vi "Remove_Child_Panel.vi"(8 "error in (no error)":errorcluster, 10 "Child_Panel in":refnum<class "Panel_Adaptive.lvclass">, 11 "Parent_Panel in":refnum<class "Panel2.lvclass">) -> (0 "error out":errorcluster, 1 "Status":bool, 2 "Child_Panel out":refnum<class "Panel_Interface.lvclass">[](array[class]), 3 "Parent_Panel out":refnum<class "Panel2.lvclass">, 4 "Child_Panel#":u32)   [LabVIEW 2021, in "Panel2.lvclass"]
uses:
  Panel2.lvclass
  C:/Program Files (x86)/Hyper State Machine Framework/SSW_Panel_Adaptive.lvlibp/Panel_Interface/Panel_Interface.lvclass
  C:/Program Files (x86)/Hyper State Machine Framework/SSW_Panel_Adaptive.lvlibp/Panel_Adaptive/Panel_Adaptive.lvclass
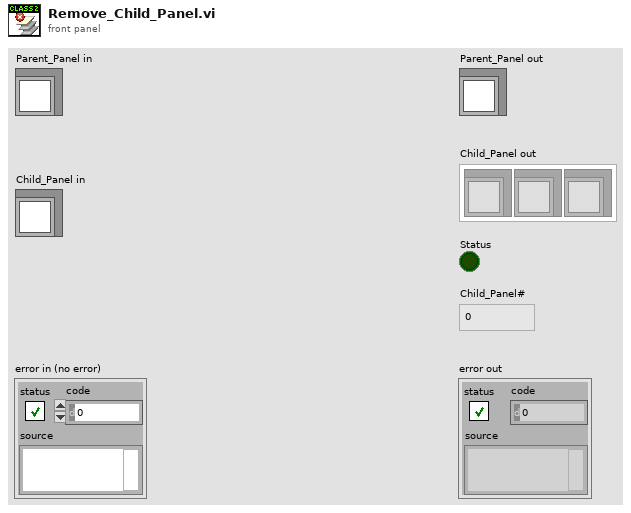
[diagram p1: front panel]
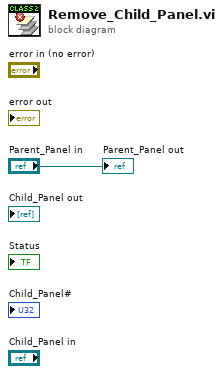
[diagram p0: block diagram]
diagram:
  "Parent_Panel out" <- "Parent_Panel in"
